vi "cRIO Main.vi"() -> ()   [LabVIEW 2017]
doc: "This application launches and executes the Tag Bus Data framework configuration for the specified target alias. This is a simple example of the framework API functions, but may also be a suitable starting point for a Host UI or Thick Client that is running a local version of the framework."
uses:
  <vilib>/NI/Module Execution Interface/Engine Runtime/Execution States.ctl
  <vilib>/NI/Module Execution Interface/Engine Runtime/Fault.ctl
  <vilib>/NI/Tag Bus Module Framework/runtime/error classification.ctl
  <vilib>/userdefined/High Color/nirio_resource_hc.ctl
  <vilib>/NI/Tag Bus Module Framework/FPGA manager/methods.ctl
  <vilib>/NI/Current Value Table/DataTypes/Double_Write.vi
  <vilib>/NI/Current Value Table/DataTypes/Double_Read.vi
  <vilib>/NI/Current Value Table/Type to Enum.vi
  <vilib>/NI/Current Value Table/DataTypes/Double_Type To Enum.vi
  <vilib>/FPGAPlugInAG/cRIO-9040/niLvFpga_Open_cRIO-9040.vi
  <vilib>/rvi/interface/common/dynamic/niFpgaDynamicAddResources.vi
  <vilib>/NI/Current Value Table/FGVs/CVT Globals.vi
  <vilib>/NI/Current Value Table/FGVs/Tag Memory.vi
  <vilib>/NI/Current Value Table/Memory Block.vi
  <vilib>/NI/Current Value Table/DataTypes/Double_Memory Block.vi
  <vilib>/rvi/interface/nirviOpenFPGA/nirviOpenFPGA.xnode
  FPGA Bitfiles/9040DCAFDemo_FPGATarget_StrainGaugeMotio_nfadPIZd4mQ.lvbitx
  <vilib>/NI/Module Execution Interface/Engine Runtime/Engine Runtime Interface.lvclass
  <vilib>/NI/DCAF/Tag Editor Core/Framework Configuration Classes/target runtime/PL_Target Runtime.lvclass
  <vilib>/NI/Tag Bus Module Framework/FPGA manager/FPGA manager.lvlib
  <vilib>/NI/Tag Bus Module Framework/runtime/TBM module execution interface.lvclass
  <vilib>/NI/Current Value Table/Current Value Table.lvlib
panel:
  in  "Value 2":dbl
  in  "Write Name 2":string
  out "Value":dbl
  in  "Read Name":string
  in  "stop 2":bool
  in  "configuration file path":path=path "/home/lvuser/NewConfigTest.pcfg"
  in  "target alias":string="cRIO"
  out "engine status":T4(array[cluster])
  in  "stop":bool
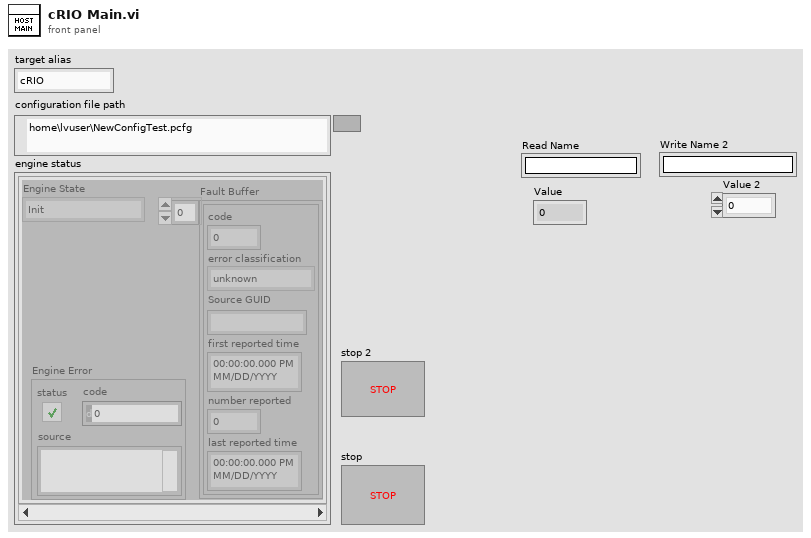
[diagram p1: front panel]
types:
  T1 = typedef "Engine Runtime Interface.lvclass/Execution States.ctl" = enum16{"Init", "Pre-Operational", "Safe-Operational", "Operational", "Stopped"}
  T2 = typedef "Engine Runtime Interface.lvclass/Fault.ctl" = cluster{"code":i32, "error classification":T3, "Source GUID":string, "first reported time":timestamp, "number reported":u32, "last reported time":timestamp}
  T3 = typedef "TBM module execution interface.lvclass/error classification.ctl" = enum16{"unknown", "none", "trivial", "recoverable", "critical"}
  T4 = cluster{"Engine State":T1, "Fault Buffer":T2[], "Engine Error":errorcluster}[]
  T5 = typedef "FPGA manager.lvlib/methods.ctl" = enum16{"initialize bitfile", "cache bitfile", "locate bitfile", "close bitfile", "clear manager"}
  T6 = typedef "nirio_resource_hc.ctl" = tag
  T7 = cluster{"Engine State":T1, "Fault Buffer":T2[], "Engine Error":errorcluster}
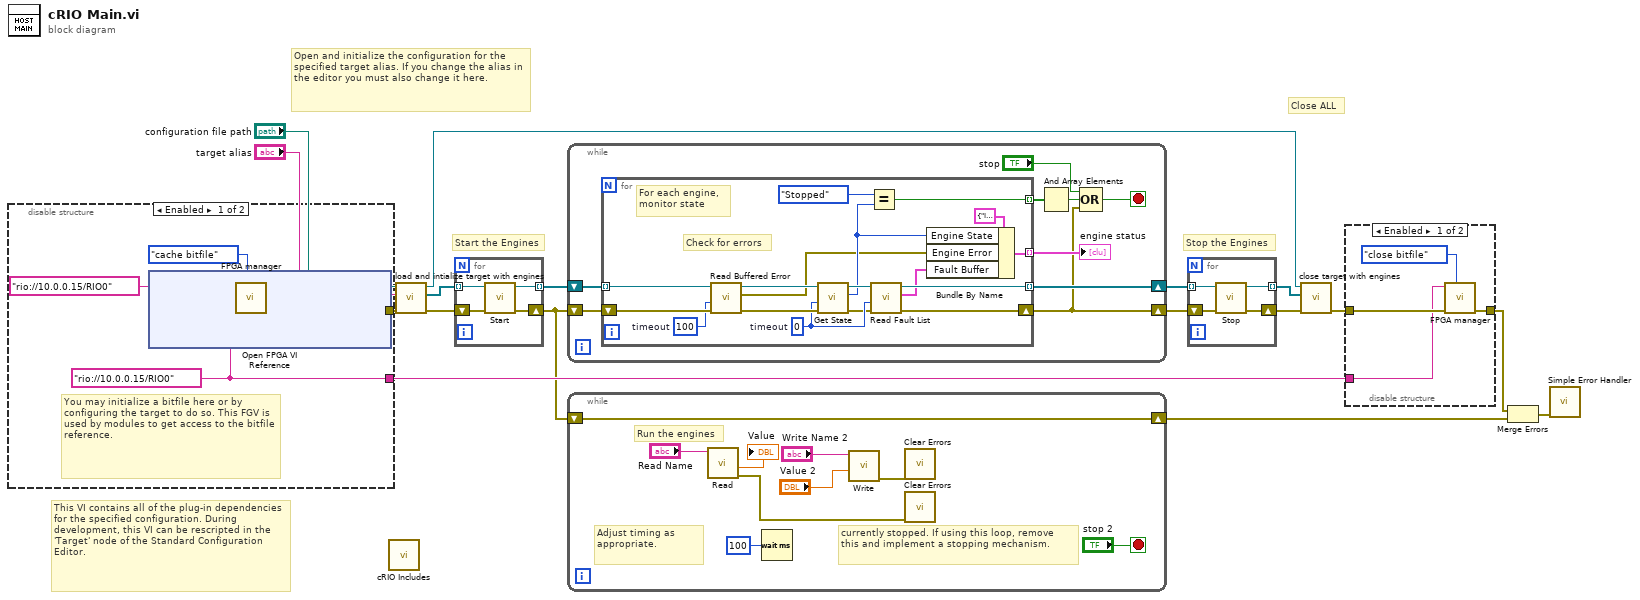
[diagram p0: block diagram]
diagram:
  # "Start the Engines"
  # "Open and initialize the configuration for the specified target alias. If you change the alias in the editor you must also change it here."
  # "Close ALL"
  # "Stop the Engines"
  # "This VI contains all of the plug-in dependencies for the specified configuration. During development, this VI can be rescripted in the 'Target' node of the Standard Configuration Editor."
  # "Run the engines"
  n1 = disable-structure shown="Enabled" {
    disable-tunnel: [w23 _] -> w7
    disable-tunnel: [w20 _] -> w6
    frame Enabled {
      w20 = T6 "rio://10.0.0.15/RIO0" ("RIO resource")
      # "You may initialize a bitfile here or by configuring the target to do so. This FGV is used by modules to get access to the bitfile reference."
      n2 = xnode "Open FPGA VI Reference"("resource name"=tag "rio://10.0.0.15/RIO0") -> ("FPGA VI Reference Out"=w22:refnum<k20>, "error out"=w18:errorcluster)  [unwired: 1 in]
      n3 = call <vilib>:"FPGA manager.vi"("action"=methods."cache bitfile", "error in"=w18, "bitfile to cache"=w22, "RIO resource"=w20) -> ("error out"=w23:errorcluster)  [unwired: 5 in, 2 out]
    }
    frame Disabled {
    }
  }
  n4 = call "cRIO Includes.vi"() -> ()  [unwired: 12 in]
  n5 = call <vilib>:"load and intialize target with engines.vi"("error in"=w7, "target alias"="target alias", "file path"="configuration file path") -> ("error out"=w14:errorcluster, "engine runtime interfaces"=w13:refnum<class "Engine Runtime Interface.lvclass">[], "target runtime"=w10:refnum<class "PL_Target Runtime.lvclass">)  [unwired: 6 in]
  n6 = for {
    tunnel: [w27] -> w17 mode=indexing
    tunnel: w13 -> [w24] mode=indexing
    shift-right: [w26] -> w5
    shift-left: w14 -> [w25]
    n7 = call-dynamic "Start.vi"("error in"=w25, "Engine Runtime Interface in"=w24) -> ("error out"=w26:errorcluster, "Engine Runtime Interface out"=w27:refnum<class "Engine Runtime Interface.lvclass">)  [unwired: 8 in]
  }
  n8 = while {
    shift-right: [w34] -> w16
    shift-left: w17 -> [w36]
    shift-right: [w28] -> w15
    shift-left: w5 -> [w35]
    stop <- w32 stop-if-true
    n9 = for {
      tunnel: w36 -> [w53] mode=indexing
      tunnel: [w45] -> w34 mode=indexing
      tunnel: [w48] -> w30 mode=indexing
      shift-right: [w44] -> w28
      shift-left: w35 -> [w52]
      tunnel: [w40] -> w31 mode=indexing
      w43 = 0  # timeout
      w47 = 100  # timeout
      # "For each engine, \nmonitor state"
      # "Check for errors"
      n10 = call-dynamic "Read Buffered Error.vi"("error in"=w52, "timeout in ms (0)"=w47, "Engine Runtime Interface in"=w53) -> ("error out"=w50:errorcluster, "Engine Error"=w38:errorcluster, "Engine Runtime Interface out"=w51:refnum<class "Engine Runtime Interface.lvclass">)  [unwired: 6 in]
      n11 = call-dynamic "Get State.vi"("error in"=w50, "timeout (-1)"=w43, "Engine Runtime Interface in"=w51) -> ("error out"=w37:errorcluster, "Engine State"=w42:T1, "Engine Runtime Interface out"=w46:refnum<class "Engine Runtime Interface.lvclass">)  [unwired: 6 in]
      n12 = Equal?(x=Execution_States."Stopped" ("Engine State"), y=w42) -> (x = y?=w48:bool)
      n13 = call-dynamic "Read Fault List.vi"("error in"=w37, "timeout (-1)"=w43, "Engine Runtime Interface in"=w46) -> ("error out"=w44:errorcluster, "faults"=w41:T2[], "Engine Runtime Interface out"=w45:refnum<class "Engine Runtime Interface.lvclass">)  [unwired: 6 in]
      n14 = Bundle By Name(cluster=T7 {"Engine State"=enum."Init", "Fault Buffer"=[], "Engine Error"={"status"=FALSE, "code"=0, "source"=""}}, "Engine State"=w42, "Engine Error"=w38, "Fault Buffer"=w41) -> (w40:T7)
    }
    "engine status" <- w31
    n15 = And Array Elements(Boolean array=w30) -> (logical AND=w29:bool)
    n16 = Compound Arithmetic op=OR("stop", w29, w28) -> (w32:bool)
  }
  n17 = while {
    shift-right: [w61] -> w4
    shift-left: w5 -> [w61]
    stop <- "stop 2" stop-if-true
    # "currently stopped. If using this loop, remove \nthis and implement a stopping mechanism."
    # "Adjust timing as appropriate."
    n18 = call-poly <vilib>:"Read.vi"("Tag Name"="Read Name") -> ("error out"=w54:errorcluster, "Value"=→"Value":dbl)  [unwired: 9 in]
    n19 = Wait (ms)(milliseconds to wait=u32 100) -> ()  [unwired: 1 out]
    n20 = call-poly <vilib>:"Write.vi"("Value"="Value 2", "Tag Name"="Write Name 2") -> ("error out"=w55:errorcluster)  [unwired: 9 in]
    n21 = call <vilib>:"Clear Errors.vi"("error in (no error)"=w55) -> ()  [unwired: 5 in, 2 out]
    n22 = call <vilib>:"Clear Errors.vi"("error in (no error)"=w54) -> ()  [unwired: 5 in, 2 out]
  }
  n23 = for {
    tunnel: w16 -> [w66] mode=indexing
    shift-right: [w63] -> w9
    shift-left: w15 -> [w65]
    tunnel: [w64] -> w11 mode=indexing
    n24 = call-dynamic "Stop.vi"("error in"=w65, "Engine Runtime Interface in"=w66) -> ("error out"=w63:errorcluster, "Engine Runtime Interface out"=w64:refnum<class "Engine Runtime Interface.lvclass">)  [unwired: 8 in]
  }
  n25 = call <vilib>:"close target with engines.vi"("error in"=w9, "Engine Runtime Interfaces"=w11, "Target Runtime"=w10) -> ("error out"=w3:errorcluster)  [unwired: 8 in]
  n26 = disable-structure shown="Enabled" {
    disable-tunnel: [w69 w71] -> w2
    disable-tunnel: w3 -> [w70 w71]
    disable-tunnel: w6 -> [w67 _]
    frame Enabled {
      n27 = call <vilib>:"FPGA manager.vi"("action"=methods."close bitfile", "error in"=w70, "RIO resource"=w67) -> ("error out"=w69:errorcluster)  [unwired: 6 in, 2 out]
    }
    frame Disabled {
    }
  }
  n28 = Merge Errors(w2, w4) -> (w1:errorcluster)
  n29 = call <vilib>:"Simple Error Handler.vi"("error in (no error)"=w1) -> ()  [unwired: 4 in, 5 out]
